vi "PowerMeterHomeMade_Graph.vi"() -> ()   [LabVIEW 2014]
uses:
  <vilib>/Analysis/baseanly.llb/Mean (DBL).vi
  <vilib>/Utility/file.llb/Write To Spreadsheet File (DBL).vi
  <vilib>/Analysis/NI_AALBase.lvlib
panel:
  in  "Escala W":dbl=0.3 format="%#_6p"
  in  "Fator Correcao":dbl=0.218 format="%#_13g"
  in  "Average Time (0.0)":dbl=1.0 format="%#_6p"
  out "Integration time (sec)":dbl=0.25 format="%#_6p"
  out "value":dbl=-0.0007075970250080372 format="%p"
  out "XY Graph 2":cluster{i32[], dbl[]}(graph)
  in  "number of samples":i32=5000
  in  "rate":dbl=20000.0
  out "Power standard deviation":dbl=0.00012941504054959165 format="%p"
  out "Power mean":dbl=0.007037856069416806 format="%p"
  out "XY Graph":cluster{i32[], dbl[]}(graph)
  in  "stop":bool
  out "Power Value":dbl=0.006926474541284404 caption="Optical Power [W]" format="%#_4p"
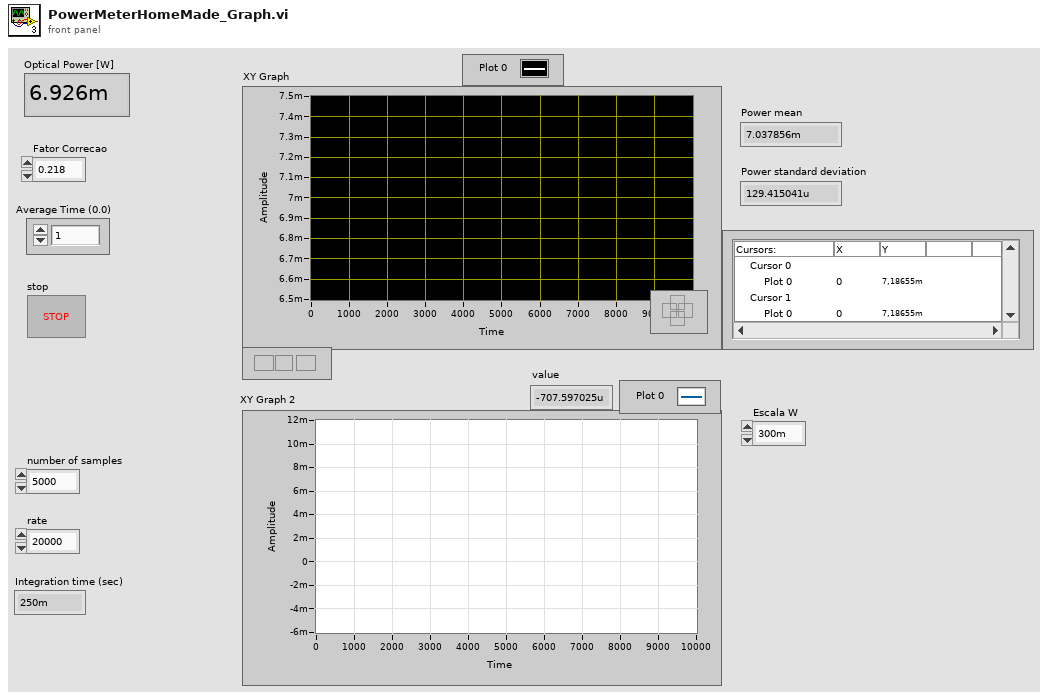
[diagram p1: front panel]
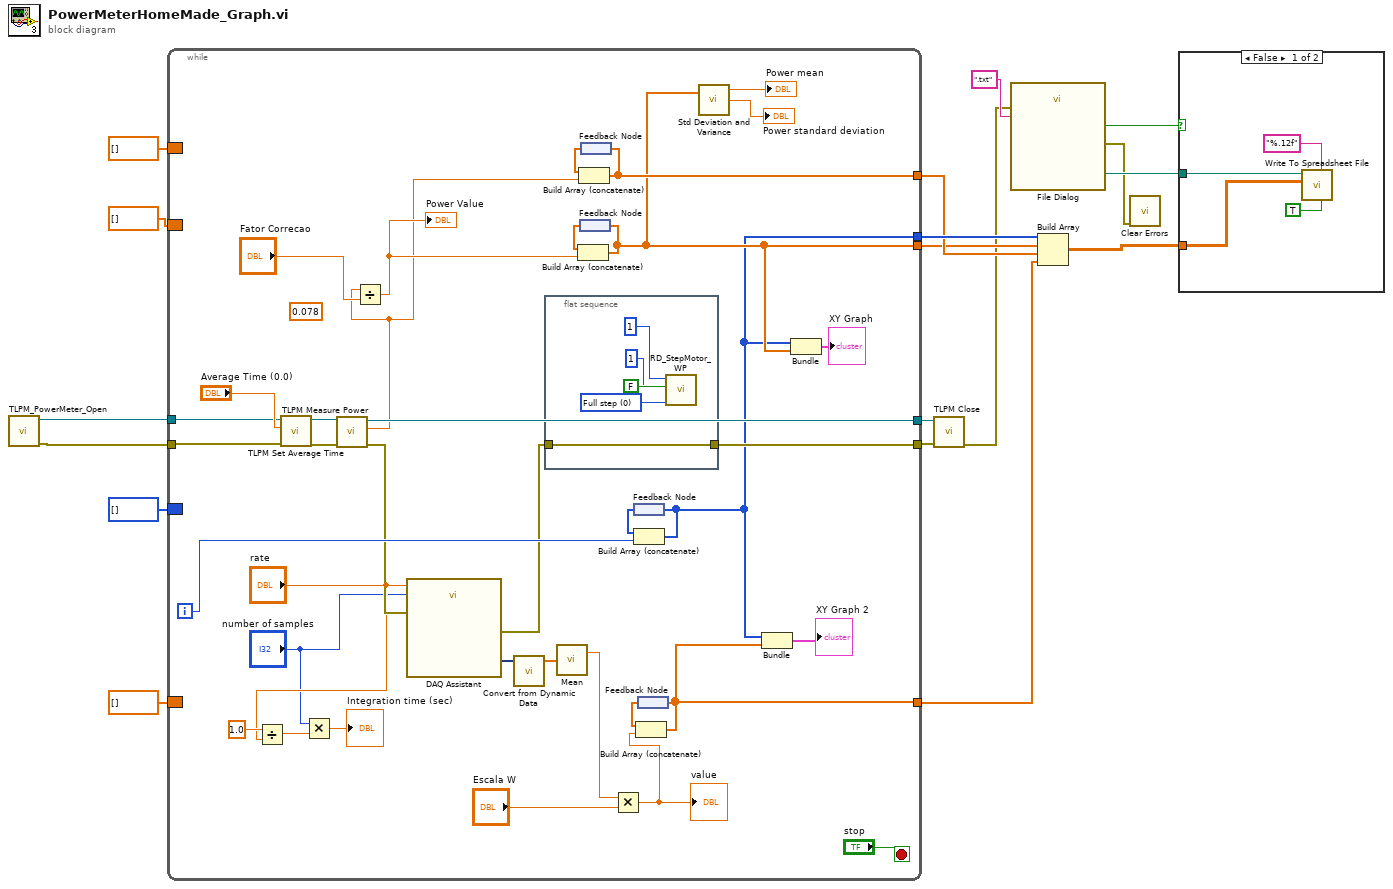
[diagram p0: block diagram]
diagram:
  n1 = call "TLPM_PowerMeter_Open.vi"() -> ("error out"=w17:errorcluster, "instrument handle out"=w18:refnum<visa-resource-name>)  [unwired: 10 in]
  n2 = while {
    tunnel: w18 -> [w25]
    tunnel: w17 -> [w26]
    tunnel: [w54] -> w16
    tunnel: [w52] -> w15
    border: i32[] [] -> [_]
    border: dbl[] [] -> [_]
    tunnel: [w43] -> w9
    tunnel: [w34] -> w12
    tunnel: [w44] -> w10
    border: dbl[] [] -> [_]
    border: dbl[] [] -> [_]
    tunnel: [w33] -> w1
    i -> [w51]
    stop <- "stop" stop-if-true
    (unwired) 0.078 ("x")
    n3 = Divide(x=1.0, y="rate") -> (x/y=w30:dbl)
    n4 = call <instrlib>:"TLPM Set Average Time.vi"("error in (no error)"=w26, "Average Time (0.0)"="Average Time (0.0)", "instrument handle"=w25) -> ("error out"=w23:errorcluster, "instrument handle out"=w24:refnum<visa-resource-name>)  [unwired: 7 in]
    n5 = Multiply(x="number of samples", y=w30) -> (x*y=→"Integration time (sec)":dbl)
    n6 = call "TLPM Measure Power.vi"("error in (no error)"=w23, "instrument handle"=w24) -> ("error out"=w40:errorcluster, "Power"=w22:dbl, "instrument handle out"=w54:refnum<visa-resource-name>)  [unwired: 7 in]
    n7 = Divide(x=w22, y="Fator Correcao") -> (x/y=w41:dbl)
    "Power Value" <- w41
    n8 = call "DAQ Assistant"("rate"="rate", "number of samples"="number of samples", "error in"=w40) -> ("data"=w38:dynamicdata, "error out"=w39:errorcluster)  [unwired: 14 in, 1 out]
    n9 = call "Convert from Dynamic Data"("Dynamic Data Type"=w38) -> ("Array"=w37:dbl[])  [unwired: 3 in]
    n10 = flat-sequence {
      tunnel: w39 -> [w59]
      tunnel: [w59] -> w52
      frame #0 {
        w58 = u16 0 items=["Full step", "Half step", "1/4 step", "1/8 step", "1/16 step", "1/32 step"] ("Step resolution")
        n11 = call "RD_StepMotor_WP.vi"("Step resolution"=w58, "Direction"=FALSE, "Time between steps (ms)"=1, "Steps"=i64 1) -> ()  [unwired: 8 in]
      }
    }
    n12 = call-poly <vilib>:"Mean.vi"("X"=w37) -> ("mean"=w20:dbl)  [unwired: 1 out]
    n13 = feedback #1() -> (w49:dbl[])
    n14 = Build Array (concatenate)(w49, w41) -> (w43:dbl[])
    n15 = feedback-in #1(w43) -> ()
    n16 = feedback #2() -> (w47:dbl[])
    n17 = Build Array (concatenate)(w47, w22) -> (w44:dbl[])
    n18 = feedback-in #2(w44) -> ()
    n19 = Multiply(x=w20, y="Escala W") -> (x*y=w19:dbl)
    "value" <- w19
    n20 = feedback #3() -> (w50:i32[])
    n21 = Build Array (concatenate)(w50, w51) -> (w34:i32[])
    n22 = feedback-in #3(w34) -> ()
    n23 = feedback #4() -> (w36:dbl[])
    n24 = Build Array (concatenate)(w36, w19) -> (w33:dbl[])
    n25 = feedback-in #4(w33) -> ()
    n26 = call <vilib>:"Std Deviation and Variance.vi"("X"=w43) -> ("mean"=→"Power mean":dbl, "standard deviation"=→"Power standard deviation":dbl)  [unwired: 1 in, 1 out]
    n27 = Bundle(w34, w33) -> (→"XY Graph 2":cluster{i32[], dbl[]})  [unwired: 1 in]
    n28 = Bundle(w34, w43) -> (→"XY Graph":cluster{i32[], dbl[]})  [unwired: 1 in]
  }
  n29 = call "TLPM Close.vi"("error in (no error)"=w15, "instrument handle"=w16) -> ("error out"=w5:errorcluster)  [unwired: 9 in]
  n30 = call "File Dialog"("error in"=w5, "pattern (all files)"=".txt") -> ("selected path"=w4:path, "cancelled"=w7:bool, "error out"=w3:errorcluster)  [unwired: 10 in, 1 out]
  n31 = Build Array(w12, w9, w10, w1) -> (w6:dbl[][])
  n32 = call <vilib>:"Clear Errors.vi"("error in (no error)"=w3) -> ()  [unwired: 5 in, 2 out]
  n33 = case shown="False" w7 {
    tunnel: w6 -> [w61 _]
    tunnel: w4 -> [w60 _]
    frame False {
      n34 = call-poly <vilib>:"Write To Spreadsheet File.vi"("transpose? (no:F)"=TRUE, "format (%.3f)"="%.12f", "2D data"=w61, "file path (dialog if empty)"=w60) -> ()  [unwired: 4 in, 1 out]
    }
    frame True {
    }
  }
